vi "Get Geocode.vi"(0 "GMaps API in":refnum<class "GMaps API.lvclass">, 5 "error in (no error)":errorcluster) -> (14 "GMaps API out":refnum<class "GMaps API.lvclass">, 15 "Geocode":cluster{"Latitude":string, "Longitude":string}, 19 "error out":errorcluster)   [LabVIEW 2016, in "GMaps API.lvclass"]
doc: "Sets converted addresses (like a street address) into geographic coordinates."
uses:
  GMaps API.lvclass
  GMaps API.lvclass/GMaps API.ctl
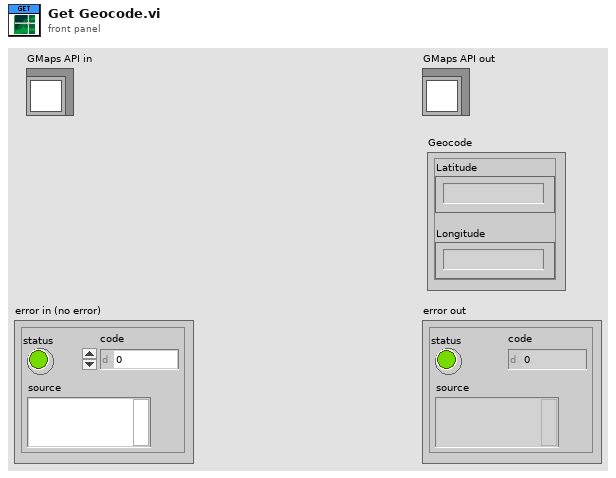
[diagram p1: front panel]
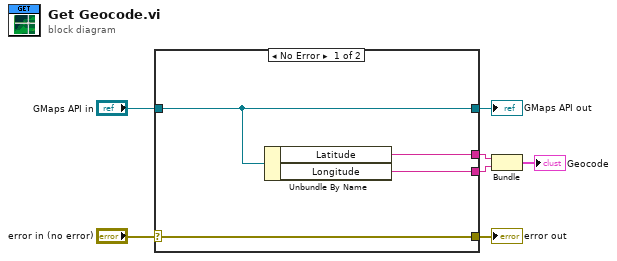
[diagram p0: block diagram]
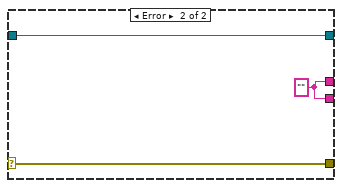
[diagram p2: hidden frame]
diagram:
  n1 = case shown="No Error" "error in (no error)" {
    selector: "error in (no error)" -> [w11 w14]
    tunnel: [w11 w14] -> w6
    tunnel: [w10 w13] -> w4
    tunnel: "GMaps API in" -> [w10 w13]
    tunnel: [w9 w12] -> w3
    tunnel: [w8 w12] -> w2
    frame No Error {
      n2 = Unbundle By Name(w10) -> ("Latitude"=w9:string, "Longitude"=w8:string)
    }
    frame Error {
      w12 = ""
    }
  }
  "error out" <- w6
  "GMaps API out" <- w4
  n3 = Bundle("Latitude"=w3, "Longitude"=w2) -> (→"Geocode":cluster{"Latitude":string, "Longitude":string})  [unwired: 1 in]
